vi "Update DatabaseA.vi"(0 "Frequency":string="40000057.37", 1 "Nominal Frequency":string, 2 "connection information":path, 3 "DC_SN":string) -> ()   [LabVIEW 2024]
uses:
  <vilib>/addons/database/Connection.llb/DB Tools Open Connec (Path).vi
  <vilib>/addons/database/Connection.llb/Conn Execute.vi
  <vilib>/addons/database/Recordset.llb/Rec Destroy - Connection.vi
  <vilib>/addons/database/_DB Variant To Data/Database Variant To Data.xnode
  <vilib>/addons/database/NI_Database_API.lvlib
panel:
  in  "Time Elapsed":dbl[](array[numeric])
  out "Time Measured":string
types:
  T1 = typedef "NI_Database_API.lvlib/Conn ObjectReference.ctl" = refnum<k1>
  T2 = typedef "NI_Database_API.lvlib/Rec ObjectReference.ctl" = refnum<k1>
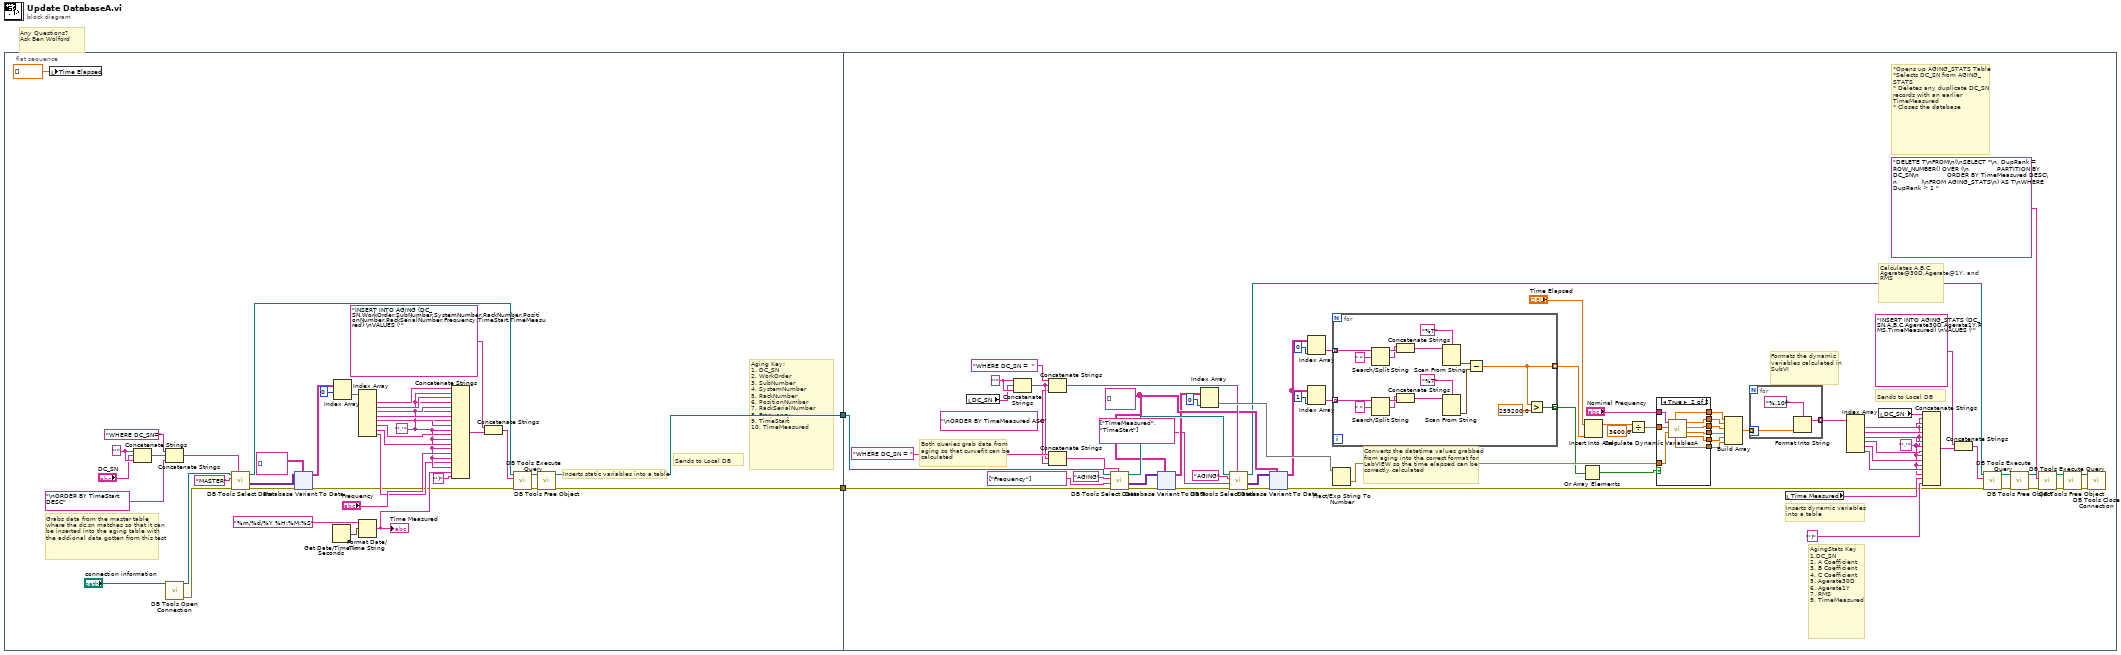
[diagram p0: block diagram]
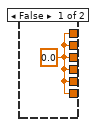
[diagram p2: hidden frame]
diagram:
  # "Any Questions?\nAsk Ben Wolford"
  n1 = flat-sequence {
    tunnel: [w4] -> w2
    tunnel: [w3] -> w1
    tunnel: w2 -> [w113]
    tunnel: w1 -> [w114]
    frame #0 {
      w22 = "'" ("string")
      w27 = "','"
      # "Grabs data from the master table where the dc.sn matches so that it can be inserted into the aging table with the addional data gotten from this test"
      # "Sends to Local DB"
      # "Inserts static variables into a table"
      # "Aging Key:\n1. DC_SN\n2. WorkOrder\n3. SubNumber\n4. SystemNumber\n5. RackNumber\n6. PositionNumber\n7. RackSerialNumber\n8. Frequency\n9. TimeStart\n10. TimeMeasured"
      n2 = local write "Time Elapsed"(dbl[] [] ("Time Elapsed")) -> ()
      n3 = Concatenate Strings(w22, "DC_SN", w22) -> (w20:string)
      n4 = Concatenate Strings("WHERE DC_SN=" ("SQL Query"), w20, "\nORDER BY TimeStart DESC" ("string")) -> (w13:string)
      n5 = call-poly <vilib>:"DB Tools Open Connection.vi"("connection information"="connection information") -> ("error out"=w17:errorcluster, "connection reference"=w18:T1)  [unwired: 7 in]
      n6 = call <vilib>:"DB Tools Select Data.vi"("condition"=w13, "error in (no error)"=w17, "table"="MASTER", "connection reference"=w18) -> ("error out"=w11:errorcluster, "data"=w15:variant[][], "connection reference out"=w7:T1)  [unwired: 2 in]
      n7 = xnode "Database Variant To Data"("database variant"=w15, "error in (no error)"=w11, "type"=string[][] [] ("table")) -> ("data"=w12:string[][], "error out"=w10:errorcluster)
      n8 = Get Date/Time In Seconds() -> (seconds since 1Jan1904=w39:timestamp)
      n9 = Index Array(array=w12, index (row)=0 ("disabled index (row)")) -> (element=w40:string[])  [unwired: 1 in]
      n10 = Index Array(array=w40) -> (element #1=w37:string, element #2=w36:string, element #3=w35:string, element #4=w34:string, element #5=w33:string, element #6=w32:string, element #7=w28:string, element #8=w24:string)  [unwired: 8 in]
      n11 = Format Date/Time String(time format string (%c)="%m/%d/%Y %H:%M:%S", seconds (now)=w39) -> (date/time string=w23:string)  [unwired: 1 in]
      "Time Measured" <- w23
      n12 = Concatenate Strings(w37, w27, w36, w27, w35, w27, w34, w27, w33, w27, w32, w27, w28, w27, "Frequency", w27, w24, w27, w23, "')" ("string")) -> (w9:string)
      n13 = Concatenate Strings("INSERT INTO AGING (DC_SN,WorkOrder,SubNumber,SystemNumber,RackNumber,PositionNumber,RackSerialNumber,Frequency,TimeStart,TimeMeasured) \nVALUES ('" ("string"), w9) -> (w8:string)
      n14 = call-poly <vilib>:"DB Tools Execute Query.vi"("error in (no error)"=w10, "SQL query"=w8, "connection reference"=w7) -> ("error out"=w5:errorcluster, "recordset reference"=w6:T2)  [unwired: 5 in]
      n15 = call-poly <vilib>:"DB Tools Free Object.vi"("error in (no error)"=w5, "recordset reference"=w6) -> ("error out"=w3:errorcluster, "connection reference"=w4:T1)  [unwired: 8 in]
    }
    frame #1 {
      w108 = string[][] [] ("SQL Query")
      w130 = "'" ("string")
      w127 = "\nORDER BY TimeMeasured ASC" ("string")
      w147 = "','" ("string")
      # "Converts the datetime values grabbed from aging into the correct format for LabVIEW so the time elapsed can be correctly calculated"
      # "Both queries grab data from aging so that curvefit can be calculated"
      # "Sends to Local DB"
      # "AgingStats Key\n1.DC_SN\n2. A Coefficient\n3. B Coefficient\n4. C Coefficient\n5. Agerate30D\n6. Agerate1Y\n7. RMS\n9. TimeMeasured"
      # "*Opens up AGING_STATS Table\n*Selects DC_SN from AGING_STATS \n* Deletes any duplicate DC_SN records with an earlier TimeMeasured\n* Closes the database"
      # "Calculates A,B,C, Agerate@30D,Agerate@1Y, and RMS"
      # "Formats the dynamic variables calculated in SubVI"
      # "Inserts dynamic variables\ninto a table"
      n16 = local read "DC_SN"() -> (w129:string)
      n17 = Concatenate Strings(w130, w129, w130) -> (w128:string)
      n18 = Concatenate Strings("WHERE DC_SN =  " ("SQL Query"), w128, w127) -> (w109:string)
      n19 = Concatenate Strings("WHERE DC_SN = " ("SQL Query"), w128, w127) -> (w115:string)
      n20 = call <vilib>:"DB Tools Select Data.vi"("condition"=w115, "error in (no error)"=w114, "columns"=string[] ["Frequency"], "table"="AGING", "connection reference"=w113) -> ("error out"=w107:errorcluster, "data"=w106:variant[][], "connection reference out"=w110:T1)  [unwired: 1 in]
      n21 = xnode "Database Variant To Data"("database variant"=w106, "error in (no error)"=w107, "type"=w108) -> ("data"=w105:string[][], "error out"=w104:errorcluster)
      n22 = Index Array(array=w105, index (col)=0 ("disabled index (col)")) -> (element=w143:string[])  [unwired: 1 in]
      n23 = call <vilib>:"DB Tools Select Data.vi"("condition"=w109, "error in (no error)"=w104, "columns"=string[] ["TimeMeasured", "TimeStart"], "table"="AGING", "connection reference"=w110) -> ("error out"=w102:errorcluster, "data"=w103:variant[][], "connection reference out"=w100:T1)  [unwired: 1 in]
      n24 = xnode "Database Variant To Data"("database variant"=w103, "error in (no error)"=w102, "type"=w108) -> ("data"=w101:string[][], "error out"=w99:errorcluster)
      n25 = Index Array(array=w101, index (col)=0 ("disabled index (col)")) -> (element=w137:string[])  [unwired: 1 in]
      n26 = Index Array(array=w101, index (col)=1 ("disabled index (col)")) -> (element=w136:string[])  [unwired: 1 in]
      n27 = for {
        tunnel: w137 -> [w266] mode=indexing
        tunnel: w136 -> [w263] mode=indexing
        tunnel: [w257] -> w135 mode=indexing
        tunnel: [w255] -> w117 mode=indexing
        n28 = Search/Split String(string=w266, search string/char (-)=" ") -> (substring before match=w260:string, match + rest of string=w258:string)  [unwired: 1 in, 1 out]
        n29 = Search/Split String(string=w263, search string/char (-)=" ") -> (substring before match=w261:string, match + rest of string=w259:string)  [unwired: 1 in, 1 out]
        n30 = Concatenate Strings(w258, w260) -> (w267:string)
        n31 = Concatenate Strings(w259, w261) -> (w262:string)
        n32 = Scan From String(format string="%T", input string=w267) -> (output 1=w269:timestamp)  [unwired: 3 in, 3 out]
        n33 = Scan From String(format string="%T", input string=w262) -> (output 1=w268:timestamp)  [unwired: 3 in, 3 out]
        n34 = Subtract(x=w269, y=w268) -> (x-y=w257:dbl)
        n35 = Greater?(x=w257, y=259200.0) -> (0:w255:bool)
      }
      n36 = Fract/Exp String To Number(string=w143) -> (number=w126:dbl[])  [unwired: 3 in, 1 out]
      n37 = Or Array Elements(Boolean array=w117) -> (logical OR=w116:bool)
      n38 = Insert Into Array(array="Time Elapsed", new element=w135) -> (w133:dbl[])  [unwired: 1 in]
      n39 = Divide(x=w133, y=3600.0) -> (x/y=w125:dbl[])
      n40 = case shown="True" w116 {
        tunnel: w126 -> [_ w254]
        tunnel: w125 -> [_ w253]
        tunnel: "Nominal Frequency" -> [_ w252]
        tunnel: [w245 w251] -> w123
        tunnel: [w245 w250] -> w122
        tunnel: [w245 w249] -> w121
        tunnel: [w245 w248] -> w120
        tunnel: [w245 w247] -> w119
        tunnel: [w245 w246] -> w118
        frame False {
          w245 = 0.0 ("Agerate30D")
        }
        frame True {
          n41 = call "Calculate Dynamic VariablesA.vi"("Frequencies"=w254, "Hours Under Test"=w253, "Nom Freq"=w252) -> ("Agerate1Y"=w251:dbl, "Agerate30D"=w250:dbl, "C"=w249:dbl, "B"=w248:dbl, "RMS"=w247:dbl, "A"=w246:dbl)  [unwired: 1 in]
        }
      }
      n42 = Build Array(w118, w120, w121, w122, w123, w119) -> (w153:dbl[])
      n43 = for {
        tunnel: w153 -> [w273] mode=indexing
        tunnel: [w272] -> w148 mode=indexing
        n44 = Format Into String(format string="%.10f", w273) -> (resulting string=w272:string)  [unwired: 2 in, 1 out]
      }
      n45 = local read "Time Measured"() -> (w132:string)
      n46 = Index Array(array=w148) -> (element #1=w150:string, element #2=w151:string, element #3=w152:string, element #4=w154:string, element #5=w155:string, element #6=w156:string)  [unwired: 6 in]
      n47 = local read "DC_SN"() -> (w140:string)
      n48 = Concatenate Strings(w140, w147, w150, w147, w151, w147, w152, w147, w154, w147, w155, w147, w156, w147, w132, "')" ("string")) -> (w149:string)
      n49 = Concatenate Strings("INSERT INTO AGING_STATS (DC_SN,A,B,C,Agerate30D,Agerate1Y,RMS,TimeMeasured) \nVALUES ('" ("string"), w149) -> (w97:string)
      n50 = call-poly <vilib>:"DB Tools Execute Query.vi"("error in (no error)"=w99, "SQL query"=w97, "connection reference"=w100) -> ("error out"=w93:errorcluster, "recordset reference"=w94:T2)  [unwired: 5 in]
      n51 = call-poly <vilib>:"DB Tools Free Object.vi"("error in (no error)"=w93, "recordset reference"=w94) -> ("error out"=w88:errorcluster, "connection reference"=w87:T1)  [unwired: 8 in]
      n52 = call-poly <vilib>:"DB Tools Execute Query.vi"("error in (no error)"=w88, "SQL query"="DELETE T\nFROM\n(\nSELECT *\n, DupRank = ROW_NUMBER() OVER (\n              PARTITION BY DC_SN\n              ORDER BY TimeMeasured DESC\n            )\nFROM AGING_STATS\n) AS T\nWHERE DupRank > 1 " ("string"), "connection reference"=w87) -> ("error out"=w89:errorcluster, "recordset reference"=w92:T2)  [unwired: 5 in]
      n53 = call-poly <vilib>:"DB Tools Free Object.vi"("error in (no error)"=w89, "recordset reference"=w92) -> ("error out"=w90:errorcluster, "connection reference"=w91:T1)  [unwired: 8 in]
      n54 = call <vilib>:"DB Tools Close Connection.vi"("error in (no error)"=w90, "connection reference"=w91) -> ()  [unwired: 5 in, 1 out]
    }
  }
